vi "CheckCollide.vi"(3 "Rectangle2":T1, 5 "Rectangle1":T1) -> (1 "Collide":bool)   [LabVIEW 2022 SP3]
panel:
  in  "IntensityArray_IN":u8[][](array[numeric])
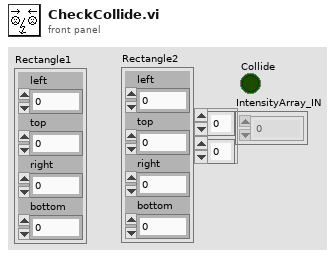
[diagram p1: front panel]
types:
  T1 = cluster{"left":i16, "top":i16, "right":i16, "bottom":i16}
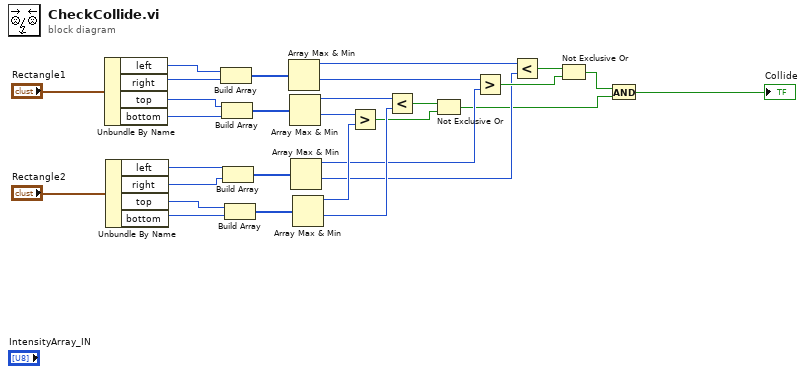
[diagram p0: block diagram]
diagram:
  n1 = Unbundle By Name("Rectangle1") -> ("left"=w16:i16, "right"=w15:i16, "top"=w29:i16, "bottom"=w28:i16)
  n2 = Unbundle By Name("Rectangle2") -> ("left"=w13:i16, "right"=w12:i16, "top"=w25:i16, "bottom"=w24:i16)
  n3 = Build Array(w16, w15) -> (w17:i16[])
  n4 = Build Array(w29, w28) -> (w27:i16[])
  n5 = Build Array(w13, w12) -> (w14:i16[])
  n6 = Build Array(w25, w24) -> (w26:i16[])
  n7 = Array Max & Min(array=w17) -> (max value=w9:i16, min value=w7:i16)  [unwired: 2 out]
  n8 = Array Max & Min(array=w27) -> (max value=w21:i16, min value=w23:i16)  [unwired: 2 out]
  n9 = Array Max & Min(array=w14) -> (max value=w6:i16, min value=w8:i16)  [unwired: 2 out]
  n10 = Array Max & Min(array=w26) -> (max value=w22:i16, min value=w20:i16)  [unwired: 2 out]
  n11 = Greater?(x=w23, y=w22) -> (0:w18:bool)
  n12 = Less?(x=w21, y=w20) -> (x < y?=w19:bool)
  n13 = Not Exclusive Or(1:w18, 2:w19) -> (0:w5:bool)
  n14 = Greater?(x=w7, y=w6) -> (0:w11:bool)
  n15 = Less?(x=w9, y=w8) -> (x < y?=w10:bool)
  n16 = Not Exclusive Or(1:w11, 2:w10) -> (0:w4:bool)
  n17 = And(x=w4, y=w5) -> (x .and. y?=→"Collide":bool)
